vi "ExportMeasuresToPDF.vi"(8 "error in (no error)":errorcluster, 11 "Table in":refnum<vi>) -> (0 "error out":errorcluster)   [LabVIEW 2012]
uses:
  Utils/Exaprom PDF/Controls/Paragraphe cluster.ctl
  Utils/Exaprom PDF/Controls/Texte alignement.ctl
  Utils/Exaprom PDF/Controls/Line spacing.ctl
  Utils/Exaprom PDF/Controls/PDF Details.ctl
  Utils/Exaprom PDF/Controls/Image or Table Caption.ctl
  Utils/Exaprom PDF/Controls/Font cluster.ctl
  Utils/Exaprom PDF/Controls/Font size.ctl
  Utils/Exaprom PDF/Controls/Font color.ctl
  Utils/Exaprom PDF/Controls/Page setup.ctl
  Utils/Exaprom PDF/Controls/Page size.ctl
  Utils/Exaprom PDF/Controls/Page Orientation.ctl
  Utils/Exaprom PDF/Controls/Page Layout Custom.ctl
  Utils/Exaprom PDF/Controls/Page margins.ctl
  GlobalVariables/UserInfos.vi
  Utils/Exaprom PDF/VIs/Text/Append Paragraph.vi
  GlobalVariables/MeasureExportStrings.vi
  GlobalVariables/MachineInfos.vi
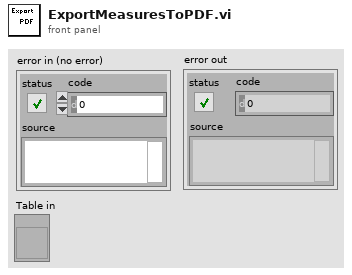
[diagram p1: front panel]
types:
  T1 = typedef "Font cluster.ctl" = cluster{"Name":string, "Size":T2, "Color":T3, "Style":cluster{"Bold":bool, "Italic":bool, "Underline":bool, "Strikeout":bool}}
  T2 = typedef "Font size.ctl" = sgl
  T3 = typedef "Font color.ctl" = u32
  T4 = typedef "Page setup.ctl" = cluster{"Page Size":T5, "Orientation":T6, "Custom Layout":T7, "Margins":T8}
  T5 = typedef "Page size.ctl" = i32
  T6 = typedef "Page Orientation.ctl" = enum16{"Portrait", "Landscape"}
  T7 = typedef "Page Layout Custom.ctl" = cluster{"Width":sgl, "Height":sgl}
  T8 = typedef "Page margins.ctl" = cluster{"Left":sgl, "Right":sgl, "Top":sgl, "Bottom":sgl}
  T9 = typedef "Paragraphe cluster.ctl" = cluster{" Aligment":T10, "Line spacing":T11}
  T10 = typedef "Texte alignement.ctl" = enum16{"Select", "CENTER", "JUSTIFY", "LEFT", "RIGHT"}
  T11 = typedef "Line spacing.ctl" = enum16{"Select", "1.0", "1.5", "2.0"}
  T12 = typedef "Image or Table Caption.ctl" = cluster{"Caption":string, "Separator":string, "Position":enum16{"Above", "Below"}}
  T13 = typedef "PDF Details.ctl" = cluster{"Title":string, "Subject":string, "Keywords":string, "Author":string, "Creator":string}
  T14 = cluster{"location":string, "Field":string, "Company":string, "Lab":string, "Operator":string, "Well":string, "Lat/Long":string, "Formation":string, "Country":string, "Client":string}
  T15 = typedef "Unit.ctl" = enum16{"inch", "mm"}
  T16 = typedef "Page dimensions.ctl" = cluster{"Start at page":i32, "Orientation":T6, "widht":sgl, "height":sgl, "Margin left":sgl, "Margin right":sgl, "Margin top":sgl, "Margin bottom":sgl}
  T17 = typedef "Header Footer [ ].ctl" = T18[]
  T18 = typedef "Header Footer cluster.ctl" = cluster{"Start page":i32, "Type":T19, "Alignment":T20, "Vertical Alignement":T21, "Image (%)":sgl, "Page #":T22, "Text":string, "Path":string, "Font":T1, "Font refnum":refnum<k24>, "Line":cluster{"Line":T23, "Thickness (points)":sgl, "Colour":T3}}
  T19 = typedef "Header Footer Type.ctl" = enum16{"Select", "Text", "Text + hyperlink", "Page number", "Image", "Image + hyperlink"}
  T20 = typedef "Header footer horiz alignment.ctl" = enum16{"Left", "Center", "Right"}
  T21 = typedef "Cell Vertical alignment.ctl" = enum16{"TOP", "MIDDLE", "BOTTOM"}
  T22 = typedef "Page number.ctl" = cluster{"Text 1":string, "Text 2":string, "Text 3":string}
  T23 = typedef "Header Footer Line.ctl" = enum16{"No line", "Horizontal line"}
  T24 = typedef "Watermark cluster2.ctl" = cluster{"Show? (F)":bool, "Type":enum16{"Image", "Text"}, "Opacity (%)":sgl, "Rotate(°)":sgl, "Position":cluster{"Position":T25, "X":sgl, "Y":sgl}, "Image path":path, "Scaled(%)":sgl, "Image refnum":refnum<k24>, "Text":string, "Font":cluster{"Name":string, "Size":T2, "Color":T3}, "Font refnum":refnum<k24>, "Alignment":T20, "Automatic":bool}
  T25 = typedef "Watermark Position.ctl" = enum16{"Absolute", "Center (page)", "Center (text section)"}
  T26 = typedef "System Fonts.ctl" = cluster{"Font name [ ]":string[], "Font and file names [ ]":cluster{"Font name":string, "File name":string}[]}
  T27 = cluster{"Document":refnum<k24>, "Writer":refnum<k24>, "Default Font":refnum<k24>, "Default Font cluster":T1, "Path":path, "Unit (default = mm)":T15, "Paragraphe cluster":T9, "Pages dimensions [ ]":T16[], "Captions":cluster{"Image":T12, "Image counter":u16, "Table":T12, "Table counter":u16, "Font":T1}, "Header":T17, "Footer":T17, "Watermark ":T24, "Actual VI name":string, "System Fonts":T26}
  T28 = cluster{"SerialNumber":string, "MachineName":string}
  T29 = cluster{"PDFTable ref":refnum<k24>, "columnWidth (points)":sgl[], "Title 1D":string[], "Table Datas 2D":string[][], "Image to Add with refnum[ ]":cluster{"Image name":string, "InstanceImage":refnum<k24>}[]}
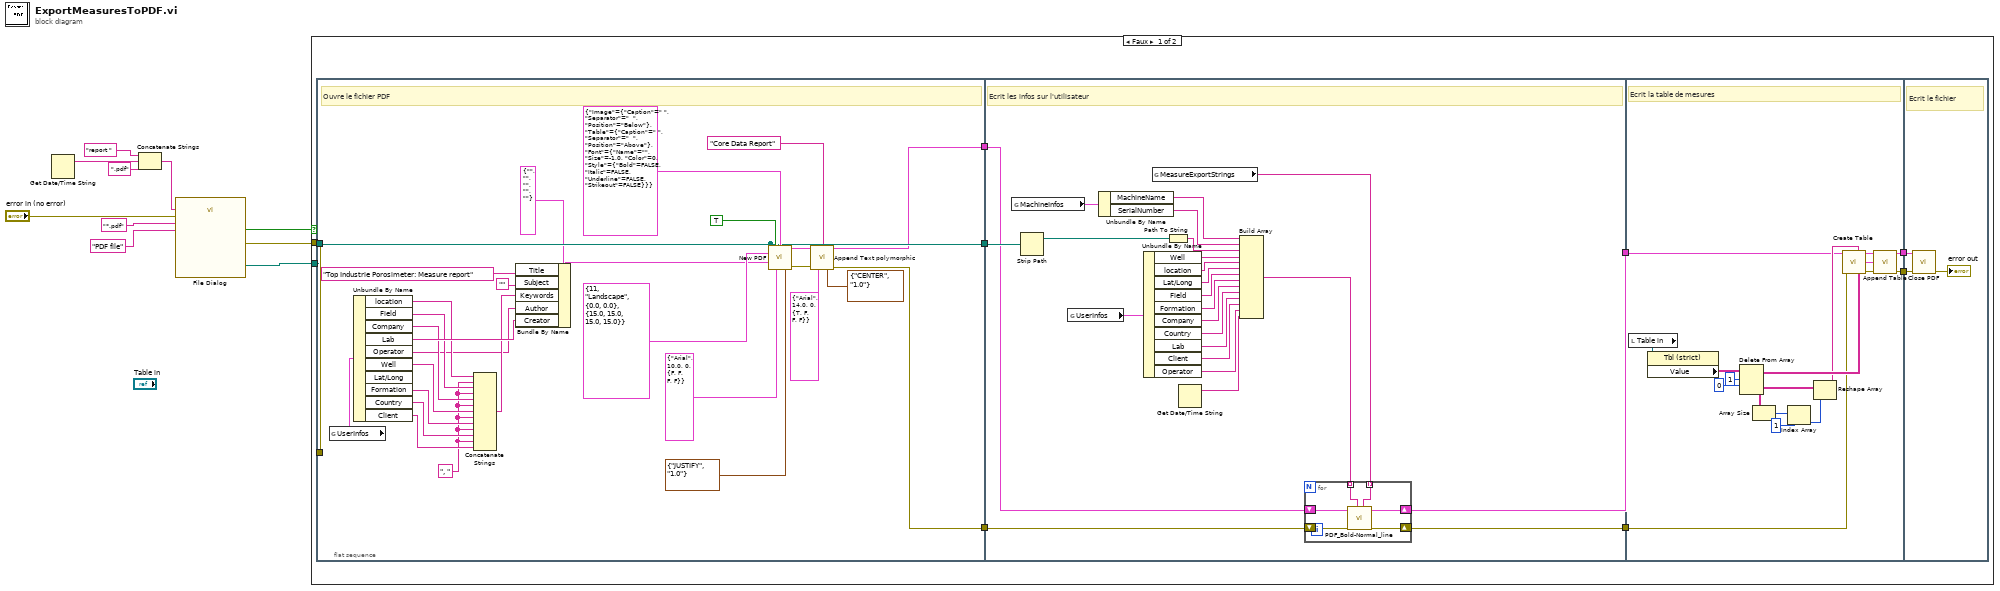
[diagram p0: block diagram]
diagram:
  n1 = Get Date/Time String() -> (date string=w2:string)  [unwired: 3 in, 1 out]
  n2 = Concatenate Strings("report " ("string"), w2, ".pdf" ("string")) -> (w3:string)
  n3 = call "File Dialog"("default name"=w3, "error in"="error in (no error)", "pattern (all files)"="*.pdf", "pattern label"="PDF file") -> ("selected path"=w6:path, "cancelled"=w1:bool, "error out"=w7:errorcluster)  [unwired: 8 in, 1 out]
  n4 = case shown="Faux" w1 {
    tunnel: w7 -> [w19 _]
    tunnel: w6 -> [w18 _]
    frame False {
      n5 = flat-sequence {
        tunnel: w19 -> [_]
        tunnel: w18 -> [w43]
        tunnel: [w43] -> w17
        tunnel: [w22] -> w16
        tunnel: [w23] -> w15
        tunnel: w17 -> [w72]
        tunnel: w16 -> [w70]
        tunnel: w15 -> [w71]
        tunnel: [w55] -> w14
        tunnel: [w54] -> w11
        tunnel: [w92] -> w13
        tunnel: w14 -> [w85]
        tunnel: [w83] -> w12
        tunnel: w11 -> [w84]
        tunnel: w13 -> [w97]
        tunnel: w12 -> [w96]
        frame #0 {
          w31 = ", "
          # "Ouvre le fichier PDF"
          n6 = global read "UserInfos.vi" "UserInfos"() -> (w42:T14)
          n7 = Unbundle By Name(w42) -> ("location"=w38:string, "Field"=w37:string, "Company"=w36:string, "Lab"=w41:string, "Operator"=w29:string, "Well"=w35:string, "Formation"=w34:string, "Country"=w33:string, "Client"=w32:string)  [unwired: 1 out]
          n8 = Concatenate Strings(w38, w31, w37, w31, w36, w31, w35, w31, w34, w31, w33, w31, w32) -> (w30:string)
          n9 = Bundle By Name(cluster=T13 {"Title"="", "Subject"="", "Keywords"="", "Author"="", "Creator"=""} ("PDF Details"), "Title"="Top Industrie Porosimeter: Measure report", "Subject"="", "Keywords"=w30, "Author"=w29, "Creator"=w41) -> (w39:T13)
          n10 = call "New PDF.vi"("PDF Path"=w43, "Overwrite?"=TRUE, "Captions"=cluster{"Image":T12, "Table":T12, "Font":T1} {"Image"={"Caption"=" ", "Separator"="  ", "Position"=enum."Below"}, "Table"={"Caption"=" ", "Separator"="  ", "Position"=enum."Above"}, "Font"={"Name"="", "Size"=-1.0, "Color"=0, "Style"={"Bold"=FALSE, "Italic"=FALSE, "Underline"=FALSE, "Strikeout"=FALSE}}}, "Page Setup"=T4 {"Page Size"=11, "Orientation"=enum."Landscape", "Custom Layout"={"Width"=0.0, "Height"=0.0}, "Margins"={"Left"=15.0, "Right"=15.0, "Top"=15.0, "Bottom"=15.0}}, "PDF Details"=w39, "Default Font"=T1 {"Name"="Arial", "Size"=10.0, "Color"=0, "Style"={"Bold"=FALSE, "Italic"=FALSE, "Underline"=FALSE, "Strikeout"=FALSE}}, "Default Paragraph"=T9 {" Aligment"=enum."JUSTIFY", "Line spacing"=enum."1.0"}) -> ("PDF Report"=w26:T27, "error out"=w25:errorcluster)  [unwired: 1 in, 6 out]
          n11 = call-poly "Append Text polymorphic.vi"("PDF Report"=w26, "Text"="Core Data Report", "error in (no error)"=w25, "Font"=T1 {"Name"="Arial", "Size"=14.0, "Color"=0, "Style"={"Bold"=TRUE, "Italic"=FALSE, "Underline"=FALSE, "Strikeout"=FALSE}}, "Paragraph properties"=T9 {" Aligment"=enum."CENTER", "Line spacing"=enum."1.0"}) -> ("PDF Report duplicate"=w22:T27, "error out"=w23:errorcluster)  [unwired: 9 in]
        }
        frame #1 {
          # "Ecrit les infos sur l'utilisateur"
          n12 = global read "MachineInfos.vi" "MachineInfos"() -> (w51:T28)
          n13 = Strip Path(path=w72) -> (stripped path=w56:path)  [unwired: 1 out]
          n14 = global read "UserInfos.vi" "UserInfos"() -> (w69:T14)
          n15 = Unbundle By Name(w51) -> ("MachineName"=w50:string, "SerialNumber"=w49:string)
          n16 = Unbundle By Name(w69) -> ("Well"=w68:string, "location"=w67:string, "Lat/Long"=w66:string, "Field"=w65:string, "Formation"=w64:string, "Company"=w61:string, "Country"=w63:string, "Lab"=w62:string, "Client"=w60:string, "Operator"=w59:string)
          n17 = global read "MeasureExportStrings.vi" "MeasureExportStrings"() -> (w53:string[])
          n18 = Path To String(path=w56) -> (string=w58:string)
          n19 = Get Date/Time String() -> (date string=w57:string)  [unwired: 3 in, 1 out]
          n20 = Build Array(w50, w49, w58, w68, w67, w66, w65, w64, w61, w63, w62, w60, w59, w57) -> (w52:string[])
          n21 = for {
            shift-right: [w76] -> w55
            shift-left: w70 -> [w77]
            shift-right: [w75] -> w54
            shift-left: w71 -> [w78]
            tunnel: w53 -> [w74] mode=indexing
            tunnel: w52 -> [w73] mode=indexing
            n22 = call "PDF_Bold-Normal_line.vi"("Bold header"=w74, "Normal text"=w73, "error in (no error)"=w78, "PDF Report IN"=w77) -> ("error out"=w75:errorcluster, "PDF Report duplicate"=w76:T27)  [unwired: 6 in]
          }
        }
        frame #2 {
          # "Ecrit la table de mesures"
          n23 = local read "Table in"() -> (w91:refnum<vi>)
          n24 = property on="Property Node" class="Tbl (strict)"(reference=w91) -> ("Value"=w90:string[][])  [unwired: 1 in, 2 out]
          n25 = Delete From Array(array=w90, length=1, index (row)=0) -> (deleted portion=w82:string[][], array with subset deleted=w87:string[][])  [unwired: 1 in]
          n26 = Array Size(array=w82) -> (size(s)=w81:i32[])
          n27 = Index Array(array=w81, index=1) -> (element=w79:i32)
          n28 = Reshape Array(w82, w79) -> (w86:string[])
          n29 = call "Create Table.vi"("PDF Report"=w85, "Title 1D"=w86, "error in (no error)"=w84, "Table Datas 2D"=w87) -> ("PDF Report duplicate"=w95:T27, "PDF Table"=w94:T29, "error out"=w93:errorcluster)  [unwired: 9 in]
          n30 = call "Append Table.vi"("PDF Report IN"=w95, "PDF Table"=w94, "error in (no error)"=w93) -> ("PDF Report OUT"=w92:T27, "error out"=w83:errorcluster)  [unwired: 11 in]
        }
        frame #3 {
          # "Ecrit le fichier"
          n31 = call "Close PDF.vi"("PDF Report"=w97, "error in (no error)"=w96) -> ("error out"=→"error out":errorcluster)  [unwired: 12 in, 1 out]
        }
      }
    }
    frame True {
    }
  }
